vi "Prober_ReadXYZTheta.vi"(8 "error in (no error)":errorcluster, 11 "SemiProbe in":refnum<class "SemiProbe.lvclass">) -> (0 "error out":errorcluster, 1 "Z location [µm]":i32, 2 "Y location [µm]":i32, 3 "X location [µm]":i32, 4 "Theta location [mdeg]":i32, 5 "SemiProbe out":refnum<class "SemiProbe.lvclass">)   [LabVIEW 2018, in "SemiProbe.lvclass"]
uses:
  SemiProbe.lvclass
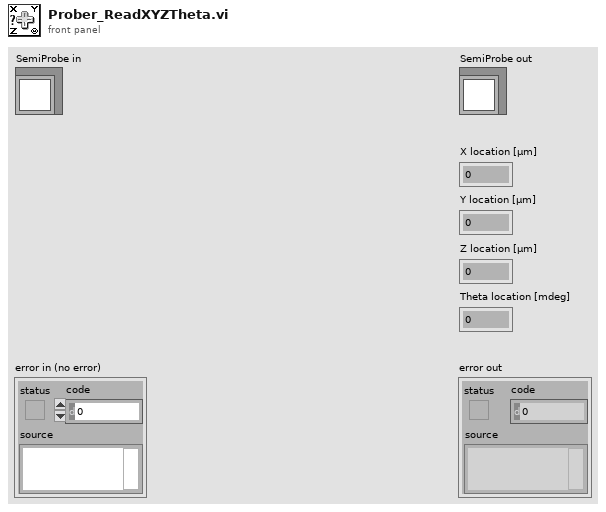
[diagram p1: front panel]
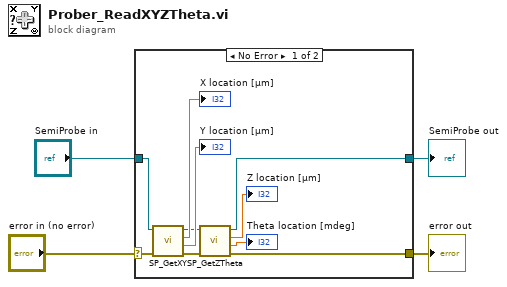
[diagram p0: block diagram]
diagram:
  n1 = case shown="No Error" "error in (no error)" {
    selector: "error in (no error)" -> [w6 w15]
    tunnel: [w9 w15] -> w3
    tunnel: [w8 w16] -> w2
    tunnel: "SemiProbe in" -> [w7 w16]
    frame No Error {
      n2 = call-dynamic "SP_GetXY.vi"("error in (no error)"=w6, "SemiProbe in"=w7) -> ("error out"=w10:errorcluster, "Y out"=→"Y location [µm]":dbl, "X out"=→"X location [µm]":dbl, "SemiProbe out"=w5:refnum<class "SemiProbe.lvclass">)  [unwired: 6 in]
      n3 = call-dynamic "SP_GetZTheta.vi"("error in (no error)"=w10, "SemiProbe in"=w5) -> ("error out"=w9:errorcluster, "Theta out [mdeg]"=→"Theta location [mdeg]":dbl, "Z out [µm]"=→"Z location [µm]":dbl, "SemiProbe out"=w8:refnum<class "SemiProbe.lvclass">)  [unwired: 6 in]
    }
    frame Error {
    }
  }
  "error out" <- w3
  "SemiProbe out" <- w2
